vi "ChangeFlag-Write.vi"(10 "ChangeFlag":u64, 11 "ChangeFlagQ":refnum<queue>) -> (2 "error out":errorcluster)   [LabVIEW 2017, in "Communicable State Machine.lvlib"]
uses:
  Communicable State Machine.lvlib
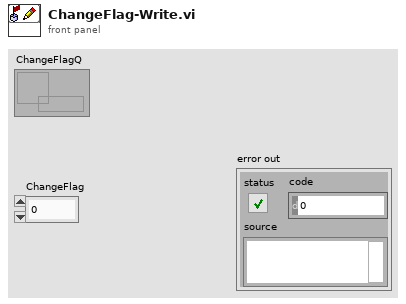
[diagram p1: front panel]
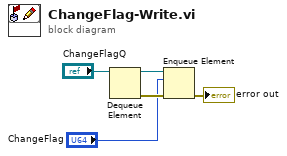
[diagram p0: block diagram]
diagram:
  n1 = Dequeue Element(queue="ChangeFlagQ") -> (queue out=w4:refnum<queue>, error out=w3:errorcluster)  [unwired: 2 in, 2 out]
  n2 = Enqueue Element(queue=w4, element="ChangeFlag", error in (no error)=w3) -> (error out=→"error out":errorcluster)  [unwired: 1 in, 2 out]
